vi "GP2Y0E03_oneshot_USB.vi"(0 "Action":u8(ring)=1 items=["Sleep", "Read"]) -> (1 "Distance (mm)":dbl format="%#.3f", 2 "Error out":errorcluster)   [LabVIEW 2014]
uses:
  Arduino_common/Arduino_comms_Global.vi
panel:
  out "read buffer":string
  out "Distance history":dbl(graph)
  out "bytes received":u32
  in  "Resource index":i32=1
  out "bytes sent":u32
  out "write buffer":string
  # "Paul Nathan, 03/10/2014"
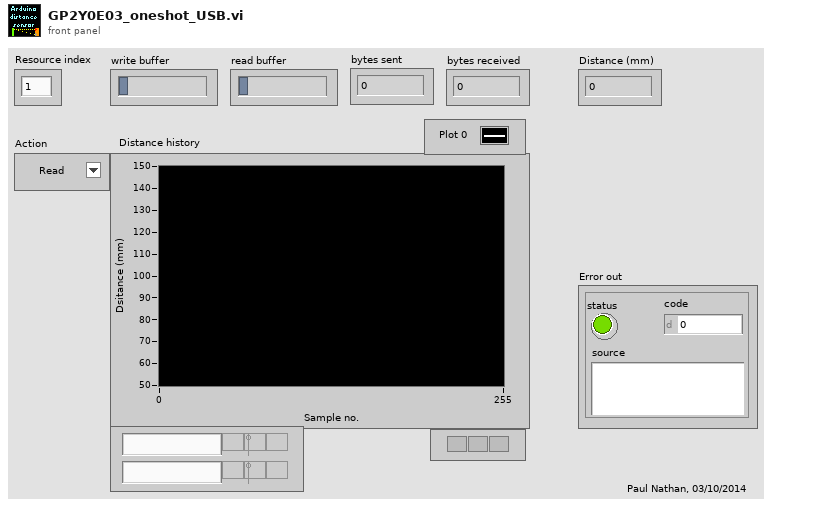
[diagram p1: front panel]
types:
  T1 = typedef "Arduino Config & resource typedef.ctl" = cluster{"VISA resource name":refnum<visa-resource-name>, "baud rate (bps)":u32, "timeout (ms)":u32, "data bits":u16, "parity":enum16{"None", "Odd", "Even", "Mark", "Space"}, "stop bits (10: 1 bit)":u16, "flow control":u16, "termination char (hex)":u8, "Enable Termination Char":bool, "byte count":u32, "Resource locked?":bool}
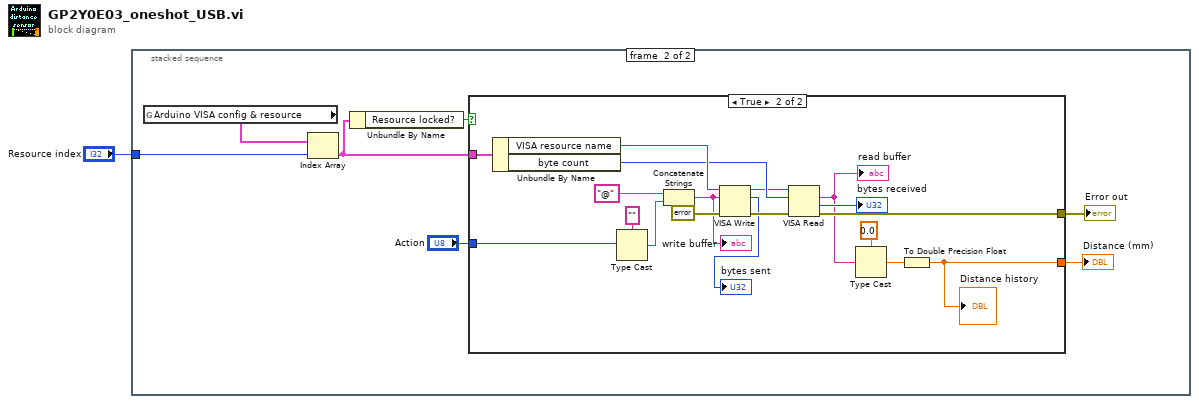
[diagram p0: block diagram]
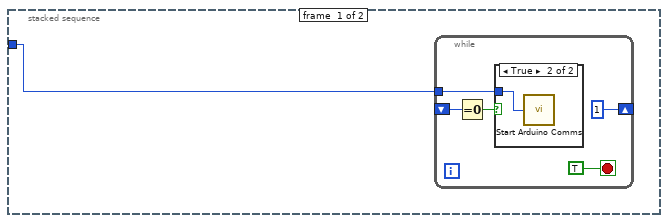
[diagram p2: hidden frame]
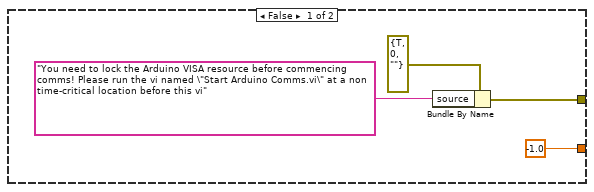
[diagram p4: hidden frame]
diagram:
  n1 = stacked-sequence {
    tunnel: "Resource index" -> [w2 w11]
    frame #0 {
      n2 = while {
        shift-right: [1] -> _
        shift-left: _ -> [w7]
        tunnel: w2 -> [w3]
        stop <- TRUE stop-if-true
        n3 = Equal To 0?(x=w7) -> (x = 0?=w6:bool)
        n4 = case shown="True" w6 {
          tunnel: w3 -> [_ w8]
          frame False {
          }
          frame True {
            n5 = call "Start Arduino Comms.vi"("Resource index"=w8) -> ()  [unwired: 1 out]
          }
        }
      }
    }
    frame #1 {
      n6 = global read "Arduino_comms_Global.vi" "Arduino VISA config & resource"() -> (w13:T1[])
      n7 = Index Array(array=w13, index=w11) -> (element=w12:T1)
      n8 = Unbundle By Name(w12) -> ("Resource locked?"=w15:bool)
      n9 = case shown="True" w15 {
        tunnel: w12 -> [_ w37]
        tunnel: [w17 w33] -> w14
        tunnel: [-1.0 w25] -> w10
        tunnel: "Action" -> [_ w24]
        frame False {
          n10 = Bundle By Name(cluster=errorcluster {"status"=TRUE, "code"=0, "source"=""} ("error out"), "source"="You need to lock the Arduino VISA resource before commencing comms! Please run the vi named \"Start Arduino Comms.vi\" at a non time-critical location before this vi") -> (w17:errorcluster)
        }
        frame True {
          n11 = Unbundle By Name(w37) -> ("VISA resource name"=w36:refnum<visa-resource-name>, "byte count"=w35:u32)
          n12 = Type Cast(type="", x=w24) -> (*(type *) &x=w22:string)
          n13 = Concatenate Strings("@", w22) -> (w20:string)
          "write buffer" <- w20
          n14 = VISA Write(VISA resource name=w36, write buffer=w20, error in (no error)=errorcluster {"status"=FALSE, "code"=0, "source"=""}) -> (VISA resource name out=w31:refnum<visa-resource-name>, return count=→"bytes sent":u32, error out=w34:errorcluster)
          n15 = VISA Read(VISA resource name=w31, byte count=w35, error in (no error)=w34) -> (read buffer=w26:string, return count=→"bytes received":u32, error out=w33:errorcluster)  [unwired: 1 out]
          "read buffer" <- w26
          n16 = Type Cast(type=sgl 0.0, x=w26) -> (*(type *) &x=w28:sgl)
          n17 = To Double Precision Float(number=w28) -> (double precision float=w25:dbl)
          "Distance history" <- w25
        }
      }
      "Error out" <- w14
      "Distance (mm)" <- w10
    }
  }
